vi "Write Config.vi"(8 "error in (no error)":errorcluster, 10 "Config":T1, 11 "Path":path) -> (0 "error out":errorcluster)   [LabVIEW 2020, in "VI Properties Editor.lvlib"]
doc: "Writes to a config file located at <B>Path</B>."
uses:
  VI Properties Editor.lvlib
  CTLs/Config.ctl
  CTLs/Filter Info.ctl
  CTLs/Filter Column.ctl
  CTLs/Filter Type.ctl
  CTLs/Config Key.ctl
  44e134d7-0004-44f8-a894-f6a922b97a70.vi
  <vilib>/Utility/config.llb/Write Key (U32).vi
  <vilib>/Utility/config.llb/Write Key (String).vi
  <vilib>/Utility/config.llb/Write Key (Boolean).vi
  <vilib>/Utility/config.llb/Write Key (I32).vi
  <vilib>/Utility/config.llb/NI_LVConfig.lvlib
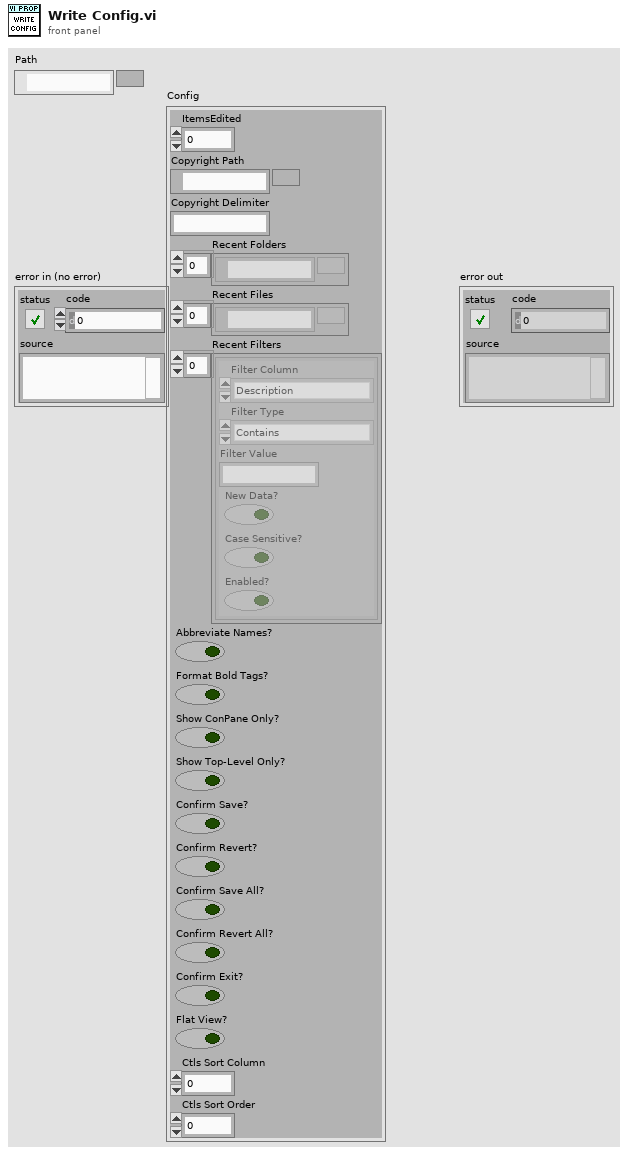
[diagram p1: front panel]
types:
  T1 = typedef "VI Properties Editor.lvlib/Config.ctl" = cluster{"ItemsEdited":u32, "Copyright Path":path, "Copyright Delimiter":string, "Recent Folders":path[], "Recent Files":path[], "Recent Filters":T2[], "Abbreviate Names?":bool, "Format Bold Tags?":bool, "Show ConPane Only?":bool, "Show Top-Level Only?":bool, "Confirm Save?":bool, "Confirm Revert?":bool, "Confirm Save All?":bool, "Confirm Revert All?":bool, "Confirm Exit?":bool, "Flat View?":bool, "Ctls Sort Column":i32, "Ctls Sort Order":i32}
  T2 = typedef "VI Properties Editor.lvlib/Filter Info.ctl" = cluster{"Filter Column":T3, "Filter Type":T4, "Filter Value":string, "New Data?":bool, "Case Sensitive?":bool, "Enabled?":bool}
  T3 = typedef "VI Properties Editor.lvlib/Filter Column.ctl" = enum16{"Name", "Path", "Type", "Window Title", "Description", "Help Path", "Help Tag", "Custom Title?", "Reentrancy", "Inlined?", "Help URL", "Help Type", "Allow Debugging?", "Auto Error Handling?", "Run When Opened?", "Suspend When Called?", "Priority", "Preferred Exec Sytem", "Control Label", "Control Caption", "Control Description", "Control Tip Strip"}
  T4 = typedef "VI Properties Editor.lvlib/Filter Type.ctl" = enum16{"Contains", "Equals", "Starts with", "Ends with", "Is empty", "Does not contain", "Does not equal", "Is not empty"}
  T5 = typedef "VI Properties Editor.lvlib/Config Key.ctl" = enum16{"ItemsEdited", "CopyrightPath", "CopyrightDelimiter", "RecentFolders", "RecentFiles", "RecentFilters", "AbbreviateNames", "ViewBold", "ShowCPCtlsOnly", "ShowTLCtlsOnly", "ConfirmSave", "ConfirmRevert", "ConfirmSaveAll", "ConfirmRevertAll", "ConfirmExit", "FlatView", "CtlsSortColumn", "CtlsSortOrder"}
  T6 = typedef "NI_LVConfig.lvlib/Config Data RefNum.ctl" = refnum<k1>
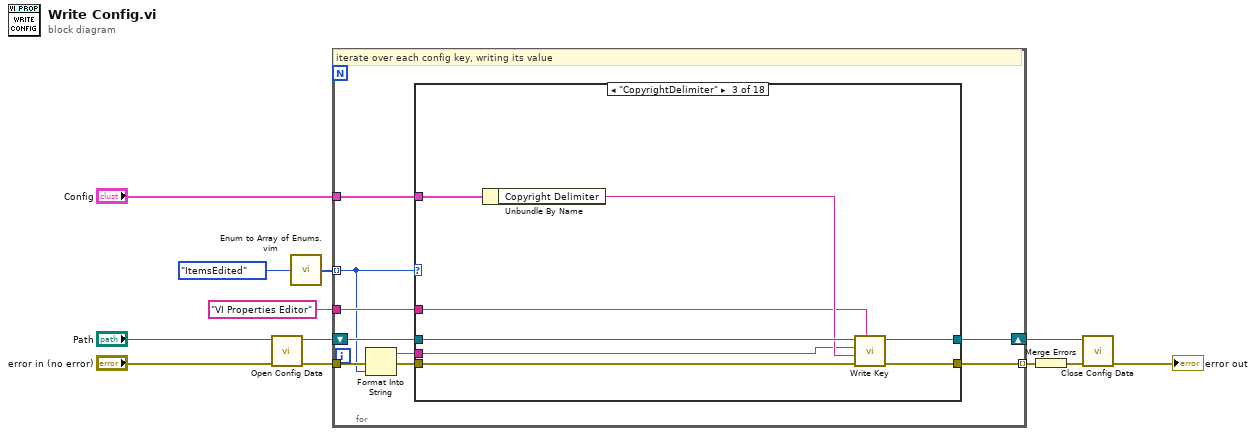
[diagram p0: block diagram]
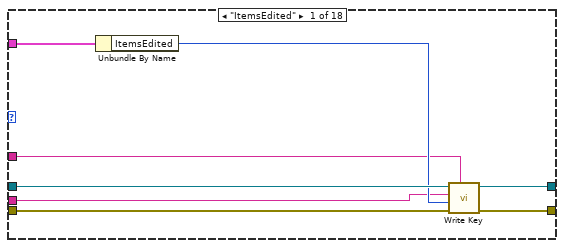
[diagram p2: hidden frame]
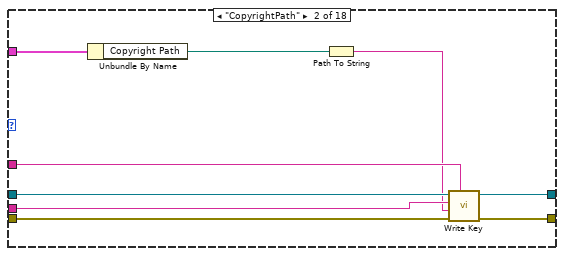
[diagram p3: hidden frame]
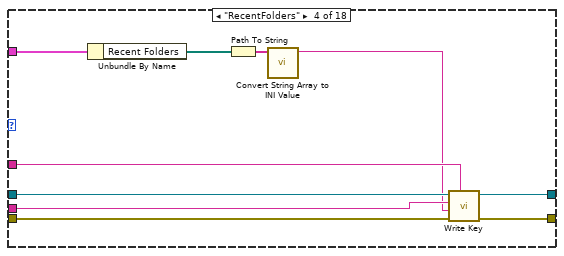
[diagram p4: hidden frame]
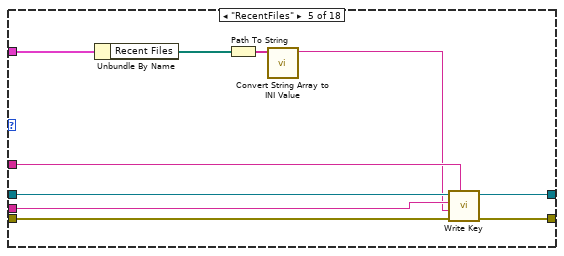
[diagram p5: hidden frame]
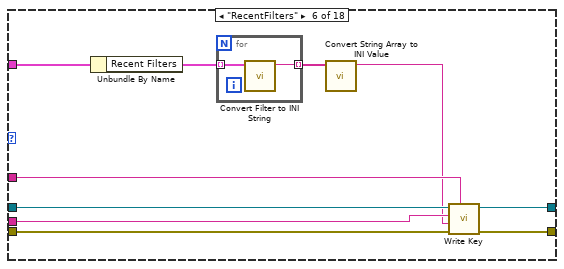
[diagram p6: hidden frame]
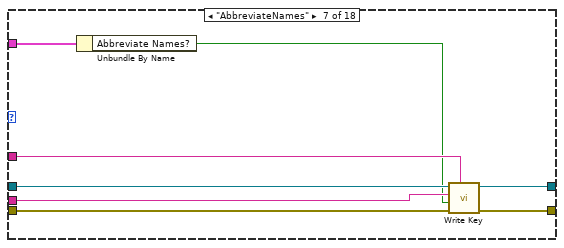
[diagram p7: hidden frame]
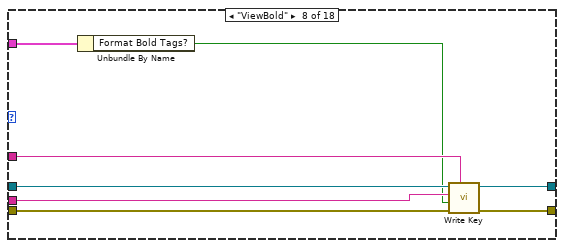
[diagram p8: hidden frame]
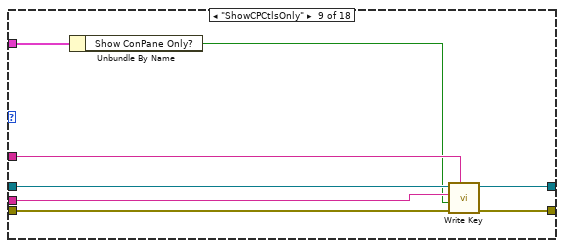
[diagram p9: hidden frame]
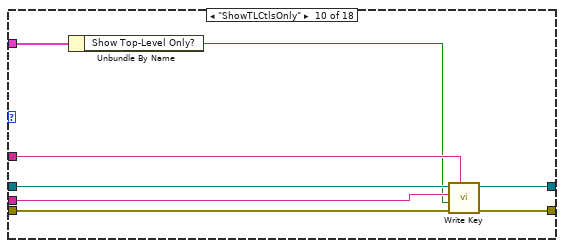
[diagram p10: hidden frame]
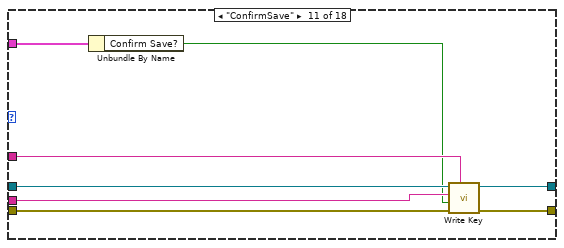
[diagram p11: hidden frame]
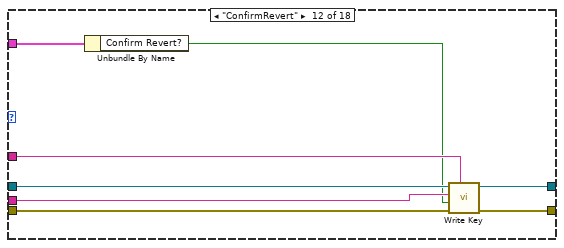
[diagram p12: hidden frame]
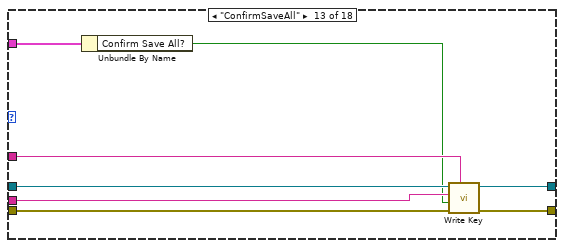
[diagram p13: hidden frame]
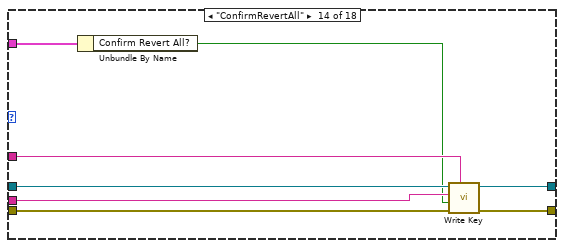
[diagram p14: hidden frame]
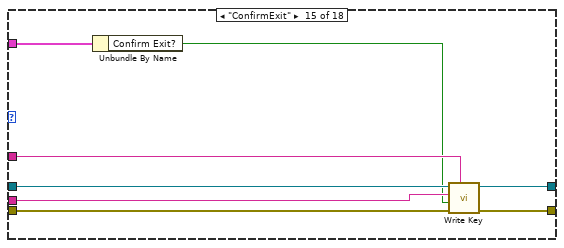
[diagram p15: hidden frame]
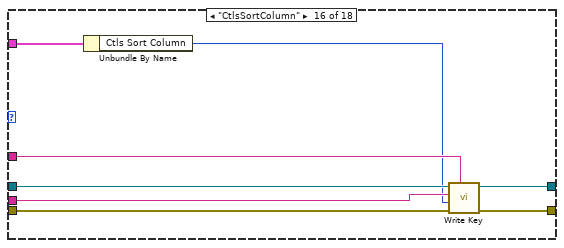
[diagram p16: hidden frame]
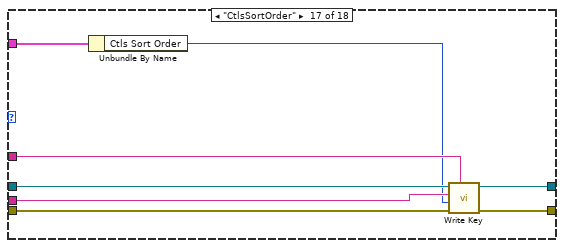
[diagram p17: hidden frame]
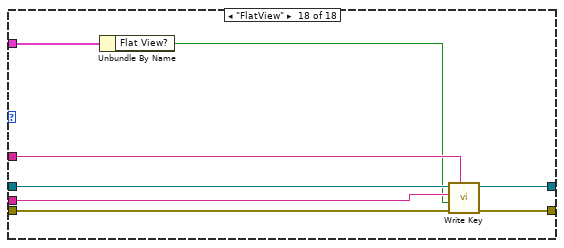
[diagram p18: hidden frame]
diagram:
  n1 = call <vilib>:"Open Config Data.vi"("error in (no error)"="error in (no error)", "configuration file path"="Path") -> ("error out"=w11:errorcluster, "refnum"=w12:T6)  [unwired: 7 in, 1 out]
  n2 = call "Enum to Array of Enums.vim"("enum"=Config_Key."ItemsEdited" ("Config Key")) -> ("array of enums"=w8:T5[])
  n3 = for {
    tunnel: w8 -> [w16] mode=indexing
    tunnel: "VI Properties Editor" ("section") -> [w17]
    tunnel: [w14] -> w6 mode=indexing
    tunnel: w11 -> [w21]
    shift-right: [w15] -> w5
    shift-left: w12 -> [w18]
    tunnel: "Config" -> [w19]
    # "iterate over each config key, writing its value"
    n4 = Format Into String(error in=w21, w16) -> (resulting string=w13:string, error out=w20:errorcluster)  [unwired: 2 in]
    n5 = case shown="\"CopyrightDelimiter\"" w16 {
      tunnel: w20 -> [w29 w38 w46 w56 w66 w76 w86 w94 w102 w110 w118 w126 w134 w142 w150 w158 w166 w174]
      tunnel: w19 -> [w27 w36 w44 w54 w64 w74 w84 w92 w100 w108 w116 w124 w132 w140 w148 w156 w164 w172]
      tunnel: w18 -> [w28 w37 w45 w55 w65 w75 w85 w93 w101 w109 w117 w125 w133 w141 w149 w157 w165 w173]
      tunnel: w17 -> [w23 w32 w40 w51 w61 w71 w81 w89 w97 w105 w113 w121 w129 w137 w145 w153 w161 w169]
      tunnel: [w26 w35 w43 w53 w63 w73 w83 w91 w99 w107 w115 w123 w131 w139 w147 w155 w163 w171] -> w15
      tunnel: [w25 w34 w42 w52 w62 w72 w82 w90 w98 w106 w114 w122 w130 w138 w146 w154 w162 w170] -> w14
      tunnel: w13 -> [w22 w31 w39 w50 w60 w70 w80 w88 w96 w104 w112 w120 w128 w136 w144 w152 w160 w168]
      frame "ItemsEdited" {
        n6 = Unbundle By Name(w27) -> ("ItemsEdited"=w24:u32)
        n7 = call-poly <vilib>:"Write Key.vi"("section"=w23, "error in (no error)"=w29, "value"=w24, "key"=w22, "refnum"=w28) -> ("error out"=w25:errorcluster, "refnum out"=w26:T6)  [unwired: 4 in, 1 out]
      }
      frame "CopyrightPath" {
        n8 = Unbundle By Name(w36) -> ("Copyright Path"=w33:path)
        n9 = Path To String(path=w33) -> (string=w30:string)
        n10 = call-poly <vilib>:"Write Key.vi"("section"=w32, "error in (no error)"=w38, "value"=w30, "key"=w31, "refnum"=w37) -> ("error out"=w34:errorcluster, "refnum out"=w35:T6)  [unwired: 4 in, 1 out]
      }
      frame "CopyrightDelimiter" {
        n11 = Unbundle By Name(w44) -> ("Copyright Delimiter"=w41:string)
        n12 = call-poly <vilib>:"Write Key.vi"("section"=w40, "error in (no error)"=w46, "value"=w41, "key"=w39, "refnum"=w45) -> ("error out"=w42:errorcluster, "refnum out"=w43:T6)  [unwired: 4 in, 1 out]
      }
      frame "RecentFolders" {
        n13 = Unbundle By Name(w54) -> ("Recent Folders"=w48:path[])
        n14 = Path To String(path=w48) -> (string=w49:string[])
        n15 = call "Convert String Array to INI Value.vi"("String Array"=w49) -> ("INI Value"=w47:string)  [unwired: 10 in]
        n16 = call-poly <vilib>:"Write Key.vi"("section"=w51, "error in (no error)"=w56, "value"=w47, "key"=w50, "refnum"=w55) -> ("error out"=w52:errorcluster, "refnum out"=w53:T6)  [unwired: 4 in, 1 out]
      }
      frame "RecentFiles" {
        n17 = Unbundle By Name(w64) -> ("Recent Files"=w58:path[])
        n18 = Path To String(path=w58) -> (string=w59:string[])
        n19 = call "Convert String Array to INI Value.vi"("String Array"=w59) -> ("INI Value"=w57:string)  [unwired: 10 in]
        n20 = call-poly <vilib>:"Write Key.vi"("section"=w61, "error in (no error)"=w66, "value"=w57, "key"=w60, "refnum"=w65) -> ("error out"=w62:errorcluster, "refnum out"=w63:T6)  [unwired: 4 in, 1 out]
      }
      frame "RecentFilters" {
        n21 = Unbundle By Name(w74) -> ("Recent Filters"=w68:T2[])
        n22 = for {
          tunnel: w68 -> [w78] mode=indexing
          tunnel: [w77] -> w69 mode=indexing
          n23 = call "Convert Filter to INI String.vi"("Filter Info"=w78) -> ("INI String"=w77:string)  [unwired: 10 in]
        }
        n24 = call "Convert String Array to INI Value.vi"("String Array"=w69) -> ("INI Value"=w67:string)  [unwired: 10 in]
        n25 = call-poly <vilib>:"Write Key.vi"("section"=w71, "error in (no error)"=w76, "value"=w67, "key"=w70, "refnum"=w75) -> ("error out"=w72:errorcluster, "refnum out"=w73:T6)  [unwired: 4 in, 1 out]
      }
      frame "AbbreviateNames" {
        n26 = Unbundle By Name(w84) -> ("Abbreviate Names?"=w79:bool)
        n27 = call-poly <vilib>:"Write Key.vi"("section"=w81, "error in (no error)"=w86, "value"=w79, "key"=w80, "refnum"=w85) -> ("error out"=w82:errorcluster, "refnum out"=w83:T6)  [unwired: 4 in, 1 out]
      }
      frame "ViewBold" {
        n28 = Unbundle By Name(w92) -> ("Format Bold Tags?"=w87:bool)
        n29 = call-poly <vilib>:"Write Key.vi"("section"=w89, "error in (no error)"=w94, "value"=w87, "key"=w88, "refnum"=w93) -> ("error out"=w90:errorcluster, "refnum out"=w91:T6)  [unwired: 4 in, 1 out]
      }
      frame "ShowCPCtlsOnly" {
        n30 = Unbundle By Name(w100) -> ("Show ConPane Only?"=w95:bool)
        n31 = call-poly <vilib>:"Write Key.vi"("section"=w97, "error in (no error)"=w102, "value"=w95, "key"=w96, "refnum"=w101) -> ("error out"=w98:errorcluster, "refnum out"=w99:T6)  [unwired: 4 in, 1 out]
      }
      frame "ShowTLCtlsOnly" {
        n32 = Unbundle By Name(w108) -> ("Show Top-Level Only?"=w103:bool)
        n33 = call-poly <vilib>:"Write Key.vi"("section"=w105, "error in (no error)"=w110, "value"=w103, "key"=w104, "refnum"=w109) -> ("error out"=w106:errorcluster, "refnum out"=w107:T6)  [unwired: 4 in, 1 out]
      }
      frame "ConfirmSave" {
        n34 = Unbundle By Name(w116) -> ("Confirm Save?"=w111:bool)
        n35 = call-poly <vilib>:"Write Key.vi"("section"=w113, "error in (no error)"=w118, "value"=w111, "key"=w112, "refnum"=w117) -> ("error out"=w114:errorcluster, "refnum out"=w115:T6)  [unwired: 4 in, 1 out]
      }
      frame "ConfirmRevert" {
        n36 = Unbundle By Name(w124) -> ("Confirm Revert?"=w119:bool)
        n37 = call-poly <vilib>:"Write Key.vi"("section"=w121, "error in (no error)"=w126, "value"=w119, "key"=w120, "refnum"=w125) -> ("error out"=w122:errorcluster, "refnum out"=w123:T6)  [unwired: 4 in, 1 out]
      }
      frame "ConfirmSaveAll" {
        n38 = Unbundle By Name(w132) -> ("Confirm Save All?"=w127:bool)
        n39 = call-poly <vilib>:"Write Key.vi"("section"=w129, "error in (no error)"=w134, "value"=w127, "key"=w128, "refnum"=w133) -> ("error out"=w130:errorcluster, "refnum out"=w131:T6)  [unwired: 4 in, 1 out]
      }
      frame "ConfirmRevertAll" {
        n40 = Unbundle By Name(w140) -> ("Confirm Revert All?"=w135:bool)
        n41 = call-poly <vilib>:"Write Key.vi"("section"=w137, "error in (no error)"=w142, "value"=w135, "key"=w136, "refnum"=w141) -> ("error out"=w138:errorcluster, "refnum out"=w139:T6)  [unwired: 4 in, 1 out]
      }
      frame "ConfirmExit" {
        n42 = Unbundle By Name(w148) -> ("Confirm Exit?"=w143:bool)
        n43 = call-poly <vilib>:"Write Key.vi"("section"=w145, "error in (no error)"=w150, "value"=w143, "key"=w144, "refnum"=w149) -> ("error out"=w146:errorcluster, "refnum out"=w147:T6)  [unwired: 4 in, 1 out]
      }
      frame "CtlsSortColumn" {
        n44 = Unbundle By Name(w156) -> ("Ctls Sort Column"=w151:i32)
        n45 = call-poly <vilib>:"Write Key.vi"("section"=w153, "error in (no error)"=w158, "value"=w151, "key"=w152, "refnum"=w157) -> ("error out"=w154:errorcluster, "refnum out"=w155:T6)  [unwired: 4 in, 1 out]
      }
      frame "CtlsSortOrder" {
        n46 = Unbundle By Name(w164) -> ("Ctls Sort Order"=w159:i32)
        n47 = call-poly <vilib>:"Write Key.vi"("section"=w161, "error in (no error)"=w166, "value"=w159, "key"=w160, "refnum"=w165) -> ("error out"=w162:errorcluster, "refnum out"=w163:T6)  [unwired: 4 in, 1 out]
      }
      frame "FlatView" {
        n48 = Unbundle By Name(w172) -> ("Flat View?"=w167:bool)
        n49 = call-poly <vilib>:"Write Key.vi"("section"=w169, "error in (no error)"=w174, "value"=w167, "key"=w168, "refnum"=w173) -> ("error out"=w170:errorcluster, "refnum out"=w171:T6)  [unwired: 4 in, 1 out]
      }
    }
  }
  n50 = Merge Errors(w6) -> (w10:errorcluster)
  n51 = call <vilib>:"Close Config Data.vi"("error in (no error)"=w10, "refnum"=w5) -> ("error out"=→"error out":errorcluster)  [unwired: 8 in, 1 out]
